vi "Get ColumnName_String_.vi"(8 "error in (no error)":errorcluster, 11 "ScriptDatabase in":refnum<class "ScriptDatabase.lvclass">) -> (0 "error out":errorcluster, 2 "ColumnName<String>":string[](array[string]), 3 "ScriptDatabase out":refnum<class "ScriptDatabase.lvclass">)   [LabVIEW 2015, in "ScriptDatabase.lvclass"]
uses:
  ScriptDatabase.lvclass
  ScriptDatabase.lvclass/ScriptDatabase.ctl
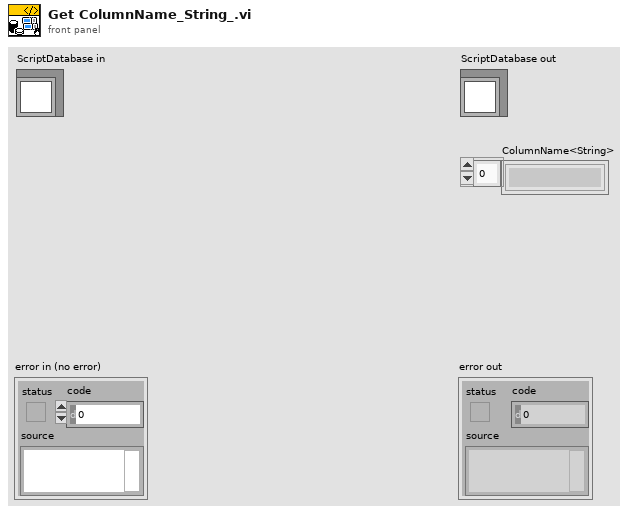
[diagram p1: front panel]
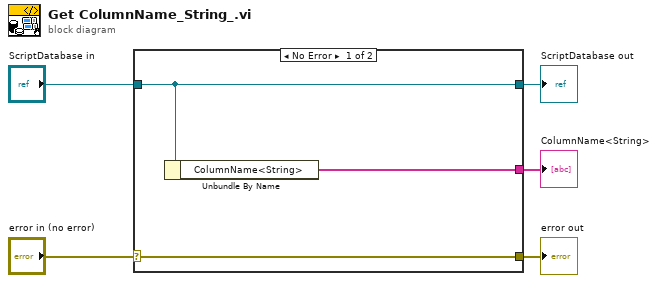
[diagram p0: block diagram]
diagram:
  n1 = case shown="No Error" "error in (no error)" {
    selector: "error in (no error)" -> [w8 w9]
    tunnel: [w8 w9] -> w4
    tunnel: [w7 w10] -> w2
    tunnel: "ScriptDatabase in" -> [w7 w10]
    tunnel: [w6 _] -> w1
    frame No Error {
      n2 = Unbundle By Name(w7) -> ("ColumnName<String>"=w6:string[])
    }
    frame Error {
    }
  }
  "error out" <- w4
  "ScriptDatabase out" <- w2
  "ColumnName<String>" <- w1
